vi "AuMT8852B EDR Max Inp Pwr Extended Test.vi"() -> ()   [LabVIEW 2017]
doc: "This example shows how to extract Extended Test Results by using multiple 'Results Panels', each configurable via the 'Stage' Configuration Input control. Note that the 'Configuration Settings' (i.e. Use Low/Medium/High Frequency), must be enabled in order to obtain valid test results in the appropriate 'Test Results' output panel."
panel:
  in  "Stage 4":T1(ring)=enum."Hop on any channels"
  out "Results 4":T2 {"3MBs Overall BER" format="%.2e"; "2MBs Overall BER" format="%.2e"}
  in  "Stage 3":T1(ring)=enum."Hop off defined high frequency"
  out "Results 3":T2 {"3MBs Overall BER" format="%.2e"; "2MBs Overall BER" format="%.2e"}
  in  "Stage 2":T1(ring)=enum."Hop off defined medium frequency"
  out "Results 2":T2 {"3MBs Overall BER" format="%.2e"; "2MBs Overall BER" format="%.2e"}
  in  "Stage":T1(ring)
  out "Results":T2 {"3MBs Overall BER" format="%.2e"; "2MBs Overall BER" format="%.2e"}
  in  "Settings":T3={"Low frequency selection"=enum."Use low frequency", "Medium frequency selection"=enum."Use medium frequency", "High frequency selection"=enum."Use high frequency", "Low TX frequency"=2480.0, "Low RX frequency"=2402.0, "Medium TX frequency"=2402.0, "Medium RX frequency"=2441.0, "High TX frequency"=2402.0, "High RX frequency"=2480.0, "Number of bits (Mbits)"=1.6, "2DHx test packet"=enum."Longest", "3DHx test packet"=enum."Longest", "Hop selection"=enum."Test with hopping off and on", "Test TX power"=-20.0, "Overall BER limit (x 1.0E-3)"=1, "Packet count"=enum."TX"} {"Test TX power" format="%.1f"; "Number of bits (Mbits)" format="%.2f"}
  out "Addresses":string[](array[string])
  in  "Start/Stop (Start)":enum16{"Start", "Stop"}(ring)
  out "error out":errorcluster
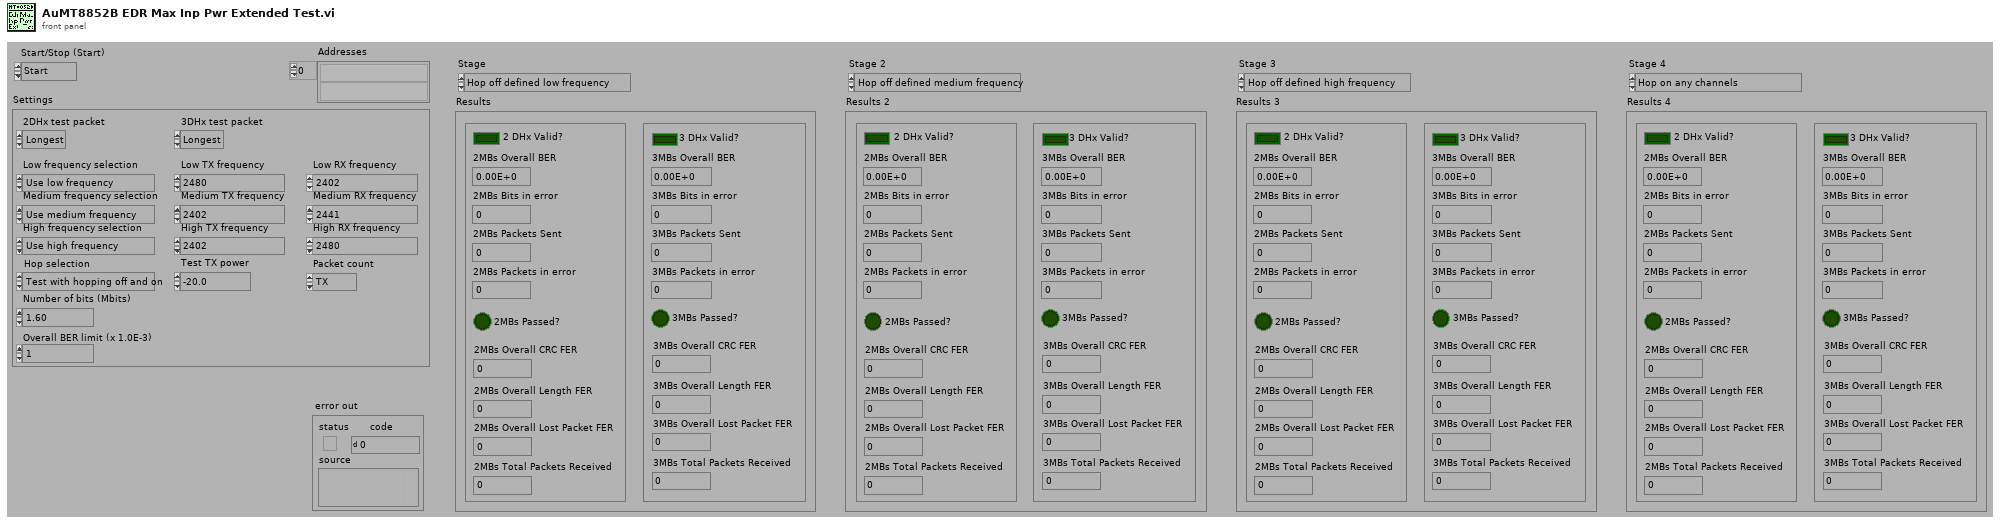
[diagram p1: front panel]
types:
  T1 = enum16{"Hop off defined low frequency", "Hop off defined medium frequency", "Hop off defined high frequency", "Hop on any channels"}
  T2 = cluster{"2 DHx Valid?":bool, "2MBs Overall BER":dbl, "2MBs Bits in error":u32, "2MBs Packets Sent":u32, "2MBs Packets in error":u32, "3 DHx Valid?":bool, "3MBs Overall BER":dbl, "3MBs Bits in error":u32, "3MBs Packets Sent":u32, "3MBs Packets in error":u32, "2MBs Overall CRC FER":u32, "2MBs Overall Length FER":u32, "2MBs Overall Lost Packet FER":u32, "3MBs Overall CRC FER":u32, "3MBs Overall Length FER":u32, "3MBs Overall Lost Packet FER":u32, "2MBs Total Packets Received":u32, "3MBs Total Packets Received":u32, "2MBs Passed?":bool, "3MBs Passed?":bool}
  T3 = cluster{"Low frequency selection":enum16{"Don't use low frequency", "Use low frequency"}, "Medium frequency selection":enum16{"Don't use medium frequency", "Use medium frequency"}, "High frequency selection":enum16{"Don't use high frequency", "Use high frequency"}, "Low TX frequency":dbl, "Low RX frequency":dbl, "Medium TX frequency":dbl, "Medium RX frequency":dbl, "High TX frequency":dbl, "High RX frequency":dbl, "Number of bits (Mbits)":dbl, "2DHx test packet":enum16{"OFF", "Longest", "2-DH1", "2-DH3", "2-DH5"}, "3DHx test packet":enum16{"OFF", "Longest", "3-DH1", "3-DH3", "3-DH5"}, "Hop selection":enum16{"Test with hopping on", "Test with hopping off", "Test with hopping off and on"}, "Test TX power":dbl, "Overall BER limit (x 1.0E-3)":i16, "Packet count":enum16{"TX", "RX"}}
  T4 = cluster{"Event status":enum16{"Event status disabled", "Event status enabled"}, "Message":enum16{"Message available disabled", "Message available enabled"}, "EUT Power State":u16, "State change":enum16{"State change disabled", "State change enabled"}, "Test failure":enum16{"Test failure disabled", "Test failure enabled"}, "Instrument status":enum16{"Instrument status disabled", "Instrument status enabled"}}
  T5 = cluster{"Completion":enum16{"Completion event disabled", "Completion event enabled"}, "Disconnect":enum16{"Disconnect event disabled", "Disconnect event enabled"}, "Connect":enum16{"Connect event disabled", "Connect event enabled"}, "Inquiry":enum16{"Inquiry event disabled", "Inquiry event enabled"}, "Temperature":enum16{"Temperature warning disabled", "Temperature warning enabled"}}
  T6 = cluster{"Reset":enum16{"Don't reset", "Reset"}, "Identity checking":enum16{"Don't query identity", "Query identity"}, "Simulation":enum16{"Don't simulate", "Simulate"}, "Range checking":enum16{"Don't check attribute ranges", "Check attribute ranges"}, "State caching":enum16{"Don't cache attributes", "Cache attributes"}, "Status checking":enum16{"Don't query instrument status", "Query instrument status"}}
  T7 = cluster{"Output power (Selected)":enum16{"Output power not selected", "Output power selected"}, "Power control (Selected)":enum16{"Power control not selected", "Power control selected"}, "Modulation index (Selected)":enum16{"Modulation index not selected", "Modulation index selected"}, "Initial carrier (Selected)":enum16{"Initial carrier not selected", "Initial carrier selected"}, "Carrier drift (Selected)":enum16{"Carrier drift not selected", "Carrier drift selected"}, "Single-slot sensitivity (Selected)":enum16{"Single-slot sensitivity not selected", "Single-slot sensitivity selected"}, "Multi-slot sensitivity (Selected)":enum16{"Multi-slot sensitivity not selected", "Multi-slot sensitivity selected"}, "Maximum input power (Selected)":enum16{"Maximum input power not selected", "Maximum input power selected"}, "Relative transmit power (Selected)":enum16{"Rel. transmit power not selected", "Rel. transmit power selected"}, "Carrier frequency stability and modulation (Selected)":enum16{"Carrier freq. and stability not selected", "Carrier freq. and stability selected"}, "Differential phase encoding":enum16{"Differential phase not selected", "Differential phase selected"}, "Sensitivity (Selected)":enum16{"Sensitivity not selected", "Sensitivity selected"}, "BER floor sensitivity (Selected)":enum16{"BER floor sensitivity not selected", "BER floor sensitivity selected"}, "EDR Maximum input power (Selected)":enum16{"EDR Max input power not selected", "EDR Max input power selected"}}
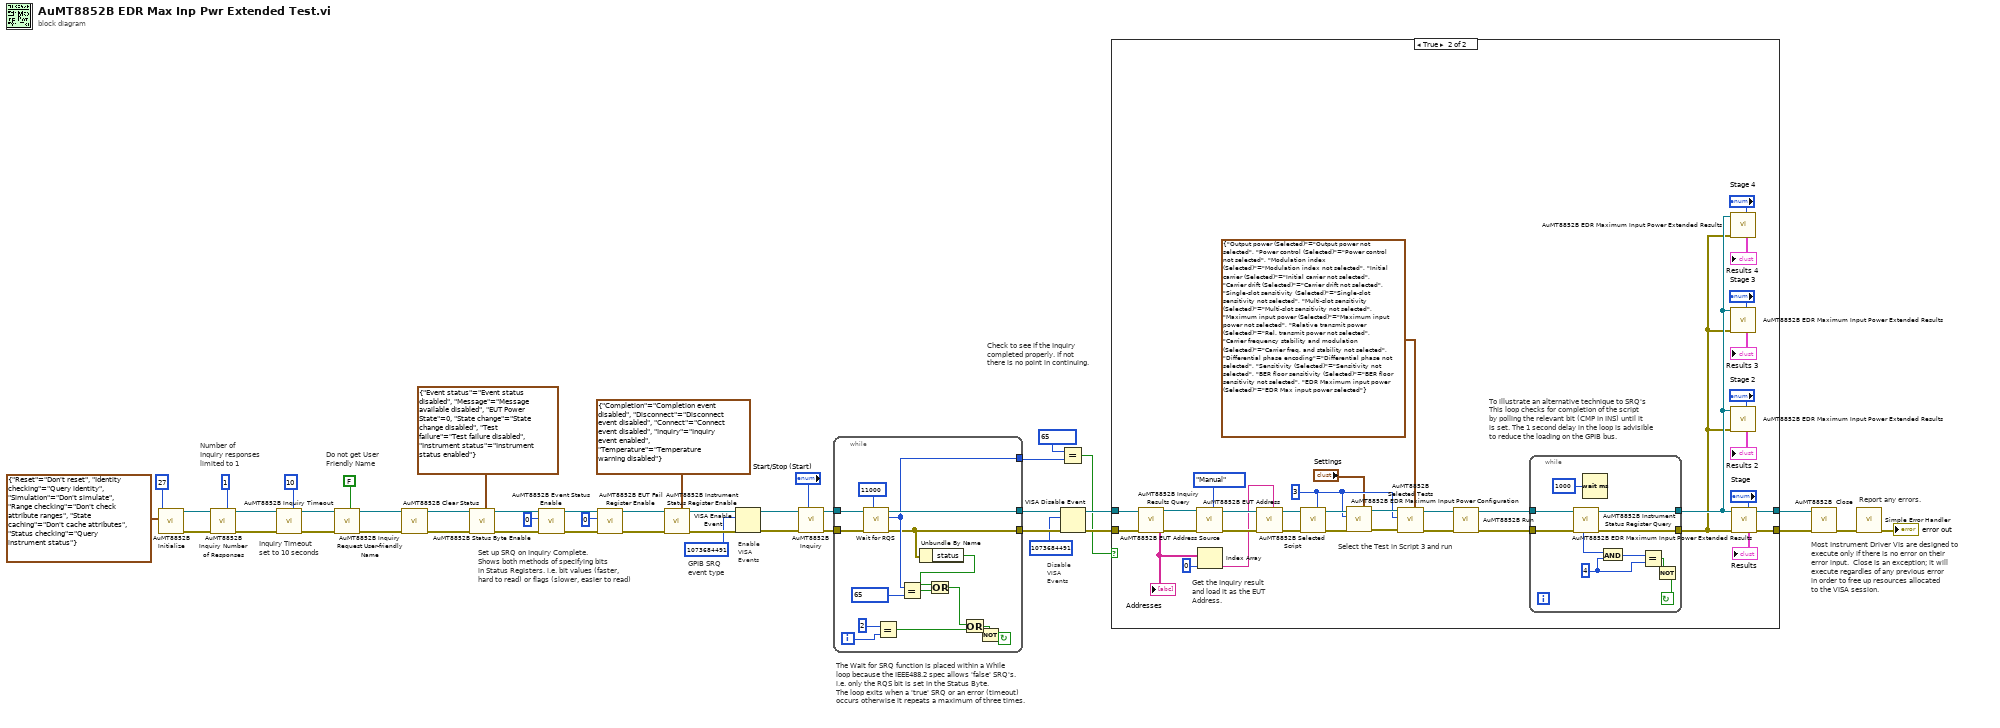
[diagram p0: block diagram]
diagram:
  # "Most Instrument Driver VIs are designed to\nexecute only if there is no error on their\nerror input.  Close is an exception; it will \nexecute regardles of any previous error\nin order to free up resources allocated\nto the VISA session."
  # "Report any errors."
  # "Check to see if the Inquiry\ncompleted properly. If not\nthere is no point in continuing."
  # "Disable\nVISA\nEvents"
  # "The Wait for SRQ function is placed within a While\nloop because the IEEE488.2 spec allows 'false' SRQ's.\ni.e. only the RQS bit is set in the Status Byte.\nThe loop exits when a 'true' SRQ or an error (timeout) \noccurs otherwise it repeats a maximum of three times."
  # "Enable\nVISA\nEvents"
  # "Set up SRQ on Inquiry Complete.\nShows both methods of specifying bits\nin Status Registers. i.e. bit values (faster, \nhard to read) or flags (slower, easier to read)"
  # "Inquiry Timeout\nset to 10 seconds"
  # "Number of\nInquiry responses\nlimited to 1"
  # "GPIB SRQ\nevent type"
  # "Do not get User\nFriendly Name"
  n1 = call <instrlib>:"AuMT8852B  Initialize.vi"("Options"=T6 {"Reset"=enum."Don't reset", "Identity checking"=enum."Query identity", "Simulation"=enum."Don't simulate", "Range checking"=enum."Don't check attribute ranges", "State caching"=enum."Don't cache attributes", "Status checking"=enum."Query instrument status"}, "GPIB Address (27)"=27) -> ("error out"=w43:errorcluster, "VISA session out"=w44:refnum<visa-resource-name>)  [unwired: 8 in]
  n2 = call <instrlib>:"AuMT8852B Inquiry Number of Responses.vi"("Responses (1)"=1, "error in (no error)"=w43, "VISA session"=w44) -> ("error out"=w41:errorcluster, "VISA session out"=w42:refnum<visa-resource-name>)  [unwired: 5 in, 2 out]
  n3 = call <instrlib>:"AuMT8852B Inquiry Timeout.vi"("Timeout (1)"=10, "error in (no error)"=w41, "VISA session"=w42) -> ("error out"=w38:errorcluster, "VISA session out"=w39:refnum<visa-resource-name>)  [unwired: 5 in, 2 out]
  n4 = call <instrlib>:"AuMT8852B Inquiry Request User-friendly Name.vi"("Status (T)"=FALSE, "error in (no error)"=w38, "VISA session"=w39) -> ("error out"=w33:errorcluster, "VISA session out"=w34:refnum<visa-resource-name>)  [unwired: 5 in, 2 out]
  n5 = call <instrlib>:"AuMT8852B Clear Status.vi"("error in (no error)"=w33, "VISA session"=w34) -> ("error out"=w31:errorcluster, "VISA session out"=w32:refnum<visa-resource-name>)  [unwired: 7 in, 1 out]
  n6 = call <instrlib>:"AuMT8852B Status Byte Enable.vi"("Flags in (all disabled)"=T4 {"Event status"=enum."Event status disabled", "Message"=enum."Message available disabled", "EUT Power State"=0, "State change"=enum."State change disabled", "Test failure"=enum."Test failure disabled", "Instrument status"=enum."Instrument status enabled"}, "error in (no error)"=w31, "VISA session"=w32) -> ("error out"=w30:errorcluster, "VISA session out"=w27:refnum<visa-resource-name>)  [unwired: 4 in, 3 out]
  n7 = call <instrlib>:"AuMT8852B Event Status Enable.vi"("error in (no error)"=w30, "Value (-1)"=0, "VISA session"=w27) -> ("error out"=w29:errorcluster, "VISA session out"=w26:refnum<visa-resource-name>)  [unwired: 4 in, 3 out]
  n8 = call <instrlib>:"AuMT8852B EUT Fail Register Enable.vi"("error in (no error)"=w29, "Value (-1)"=0, "VISA session"=w26) -> ("error out"=w28:errorcluster, "VISA session out"=w25:refnum<visa-resource-name>)  [unwired: 4 in, 3 out]
  n9 = call <instrlib>:"AuMT8852B Instrument Status Register Enable.vi"("Flags"=T5 {"Completion"=enum."Completion event disabled", "Disconnect"=enum."Disconnect event disabled", "Connect"=enum."Connect event disabled", "Inquiry"=enum."Inquiry event enabled", "Temperature"=enum."Temperature warning disabled"}, "error in (no error)"=w28, "VISA session"=w25) -> ("error out"=w20:errorcluster, "VISA session out"=w21:refnum<visa-resource-name>)  [unwired: 4 in, 3 out]
  n10 = VISA Enable Event(8:w20, 10:u32 1073684491 ("event type"), 11:w21) -> (0:w18:errorcluster, 3:w19:refnum<visa-resource-name>)  [unwired: 1 in]
  n11 = call <instrlib>:"AuMT8852B Inquiry.vi"("Start/Stop (Start)"="Start/Stop (Start)", "error in (no error)"=w18, "VISA session"=w19) -> ("error out"=w16:errorcluster, "VISA session out"=w17:refnum<visa-resource-name>)  [unwired: 6 in, 1 out]
  n12 = while {
    tunnel: w17 -> [w60]
    tunnel: w16 -> [w59]
    tunnel: [w58] -> w15
    tunnel: [w50] -> w14
    tunnel: [w51] -> w8
    i -> [w55]
    stop <- w46 continue-if-true
    n13 = call <vilib>:"Wait for RQS.VI"("timeout (25000 ms)"=u32 11000 ("timeout ms"), "error in (no error)"=w59, "VISA resource name"=w60) -> ("error out"=w50:errorcluster, "status byte"=w51:u16, "VISA resource name out"=w58:refnum<visa-resource-name>)  [unwired: 6 in]
    n14 = Equal?(x=2, y=w55) -> (x = y?=w56:bool)
    n15 = Equal?(x=w51, y=u16 65) -> (x = y?=w49:bool)
    n16 = Unbundle By Name(w50) -> ("status"=w48:bool)
    n17 = Or(x=w48, y=w49) -> (x .or. y?=w47:bool)
    n18 = Or(x=w47, y=w56) -> (x .or. y?=w57:bool)
    n19 = Not(x=w57) -> (.not. x?=w46:bool)
  }
  n20 = Equal?(x=u16 65, y=w8) -> (x = y?=w9:bool)
  n21 = VISA Disable Event(8:w14, 10:u32 1073684491 ("event type"), 11:w15) -> (0:w12:errorcluster, 3:w13:refnum<visa-resource-name>)  [unwired: 1 in]
  n22 = case shown="True" w9 {
    tunnel: [w62 w85] -> w40
    tunnel: w13 -> [w62 w97]
    tunnel: w12 -> [w61 w96]
    tunnel: [w61 w82] -> w4
    frame False {
    }
    frame True {
      w74 = 3 ("Script (3)")
      # "To illustrate an alternative technique to SRQ's\nThis loop checks for completion of the script\nby polling the relevant bit (CMP in INS) until it\nis set. The 1 second delay in the loop is advisible\nto reduce the loading on the GPIB bus."
      # "Select the Test in Script 3 and run"
      # "Get the Inquiry result\nand load it as the EUT\nAddress."
      n23 = call <instrlib>:"AuMT8852B Inquiry Results Query.vi"("error in (no error)"=w96, "VISA session"=w97) -> ("error out"=w94:errorcluster, "VISA session out"=w95:refnum<visa-resource-name>, "Addresses"=w90:string[])  [unwired: 5 in, 2 out]
      "Addresses" <- w90
      n24 = call <instrlib>:"AuMT8852B EUT Address Source.vi"("Source (Manual)"=enum16{"Manual", "RS-232", "USB", "Inquiry"}."Manual", "error in (no error)"=w94, "VISA session"=w95) -> ("error out"=w92:errorcluster, "VISA session out"=w91:refnum<visa-resource-name>)  [unwired: 5 in, 2 out]
      n25 = Index Array(array=w90, index=0 ("Index")) -> (element=w88:string)
      n26 = call <instrlib>:"AuMT8852B EUT Address.vi"("EUT Address (0x000000000000)"=w88, "error in (no error)"=w92, "VISA session"=w91) -> ("error out"=w84:errorcluster, "VISA session out"=w87:refnum<visa-resource-name>)  [unwired: 5 in, 2 out]
      n27 = call <instrlib>:"AuMT8852B Selected Script.vi"("Script (3)"=w74, "error in (no error)"=w84, "VISA session"=w87) -> ("error out"=w78:errorcluster, "VISA session out"=w76:refnum<visa-resource-name>)  [unwired: 5 in, 2 out]
      n28 = call <instrlib>:"AuMT8852B EDR Maximum Input Power Configuration.vi"("Settings"="Settings", "error in (no error)"=w78, "Script (3)"=w74, "VISA session"=w76) -> ("error out"=w77:errorcluster, "VISA session out"=w75:refnum<visa-resource-name>)  [unwired: 4 in, 2 out]
      n29 = call <instrlib>:"AuMT8852B Selected Tests.vi"("Tests (All selected)"=T7 {"Output power (Selected)"=enum."Output power not selected", "Power control (Selected)"=enum."Power control not selected", "Modulation index (Selected)"=enum."Modulation index not selected", "Initial carrier (Selected)"=enum."Initial carrier not selected", "Carrier drift (Selected)"=enum."Carrier drift not selected", "Single-slot sensitivity (Selected)"=enum."Single-slot sensitivity not selected", "Multi-slot sensitivity (Selected)"=enum."Multi-slot sensitivity not selected", "Maximum input power (Selected)"=enum."Maximum input power not selected", "Relative transmit power (Selected)"=enum."Rel. transmit power not selected", "Carrier frequency stability and modulation (Selected)"=enum."Carrier freq. and stability not selected", "Differential phase encoding"=enum."Differential phase not selected", "Sensitivity (Selected)"=enum."Sensitivity not selected", "BER floor sensitivity (Selected)"=enum."BER floor sensitivity not selected", "EDR Maximum input power (Selected)"=enum."EDR Max input power selected"}, "error in (no error)"=w77, "Script (3)"=w74, "VISA session"=w75) -> ("error out"=w83:errorcluster, "VISA session out"=w86:refnum<visa-resource-name>)  [unwired: 4 in, 2 out]
      n30 = call <instrlib>:"AuMT8852B Run.vi"("error in (no error)"=w83, "VISA session"=w86) -> ("error out"=w80:errorcluster, "VISA session out"=w81:refnum<visa-resource-name>)  [unwired: 7 in, 1 out]
      n31 = while {
        tunnel: w81 -> [w107]
        tunnel: [w106] -> w64
        tunnel: w80 -> [w105]
        tunnel: [w104] -> w63
        stop <- w98 continue-if-true
        w99 = 4 ("y")
        n32 = call <instrlib>:"AuMT8852B Instrument Status Register Query.vi"("error in (no error)"=w105, "VISA session"=w107) -> ("error out"=w104:errorcluster, "VISA session out"=w106:refnum<visa-resource-name>, "Value"=w100:i32)  [unwired: 5 in, 2 out]
        n33 = Wait (ms)(milliseconds to wait=u32 1000) -> ()  [unwired: 1 out]
        n34 = And(x=w100, y=w99) -> (x .and. y?=w101:i32)
        n35 = Equal?(x=w101, y=w99) -> (x = y?=w102:bool)
        n36 = Not(x=w102) -> (.not. x?=w98:bool)
      }
      n37 = call <instrlib>:"AuMT8852B EDR Maximum Input Power Extended Results.vi"("Stage"="Stage 4", "error in (no error)"=w63, "VISA session"=w64) -> ("Results"=→"Results 4":T2)  [unwired: 5 in, 3 out]
      n38 = call <instrlib>:"AuMT8852B EDR Maximum Input Power Extended Results.vi"("Stage"="Stage 3", "error in (no error)"=w63, "VISA session"=w64) -> ("Results"=→"Results 3":T2)  [unwired: 5 in, 3 out]
      n39 = call <instrlib>:"AuMT8852B EDR Maximum Input Power Extended Results.vi"("Stage"="Stage 2", "error in (no error)"=w63, "VISA session"=w64) -> ("Results"=→"Results 2":T2)  [unwired: 5 in, 3 out]
      n40 = call <instrlib>:"AuMT8852B EDR Maximum Input Power Extended Results.vi"("Stage"="Stage", "error in (no error)"=w63, "VISA session"=w64) -> ("error out"=w82:errorcluster, "VISA session out"=w85:refnum<visa-resource-name>, "Results"=→"Results":T2)  [unwired: 5 in, 1 out]
    }
  }
  n41 = call <instrlib>:"AuMT8852B  Close.vi"("error in (no error)"=w4, "VISA session"=w40) -> ("error out"=w2:errorcluster)  [unwired: 8 in, 1 out]
  n42 = call <vilib>:"Simple Error Handler.vi"("error in (no error)"=w2) -> ("error out"=→"error out":errorcluster)  [unwired: 4 in, 4 out]
